vi "PLC.vi"() -> ()   [LabVIEW 2016]
doc: "Sound Analyzer queued state machine"
uses:
  PLC.Data.ctl
  PLC.Data.Status.ctl
  PLC.State.ctl
  PLC.Data.Sets.ctl
  LowLevel/PLC.DataBlock.PCstatus.ctl
  LowLevel/PLC.DataBlock.PCstatus.General.ctl
  LowLevel/PLC.DataBlock.PCstatus.Station.ctl
  LowLevel/PLC.DataBlock.PLCstatus.ctl
  LowLevel/PLC.DataBlock.PLCstatus.General.ctl
  LowLevel/PLC.DataBlock.PLCstatus.Station.ctl
  PLC.Action.ctl
  Tools/CitTemplate/citTemplate.errData.ctl
  Tools/EventLog/EventLog.EventSource.ctl
  PLC.CheckStatusReassembly.ctl
  Database/Database.Global.vi
  PLC.Global.vi
panel:
  out "action":T1=enum."-- PLC --"
  out "error.action":string
  out "error":errorcluster
  out "Data":T2={"Status"={"Idx"=0, "ConnRef"=0, "State"=enum."Off", "LiveBitTimer"=timestamp(0 s since 1904-01-01)}, "Sets"={"Enable"=FALSE, "IP"="", "Rack"=0, "Slot"=10000, "LifeBitTimer_s"=0.0, "DataBlockAddr_PCStatus"=0, "DataBlockAddr_PLCStatus"=1, "DataBlockAddr_PLCNewData"=[], "DataBlockSize_PLCNewData"=[], "DataBlockAddr_PLCChangeOver"=[], "DataBlockSize_PLCChangeOver"=[], "DataBlockAddr_PCChangeOver"=[], "DataBlockAddr_PLCCheckStatus"=[], "DataBlockSize_PLCCheckStatus"=[], "DataBlockAddr_PCCheckStatus"=[]}, "PCstatus"={"General"={"LifeBit"=FALSE, "DbRun"=FALSE}, "Stations"=[]}, "PLCstatus"={"General"={"LifeBit"=FALSE}, "Stations"=[]}}
  out "_loop":i32(ring)=4
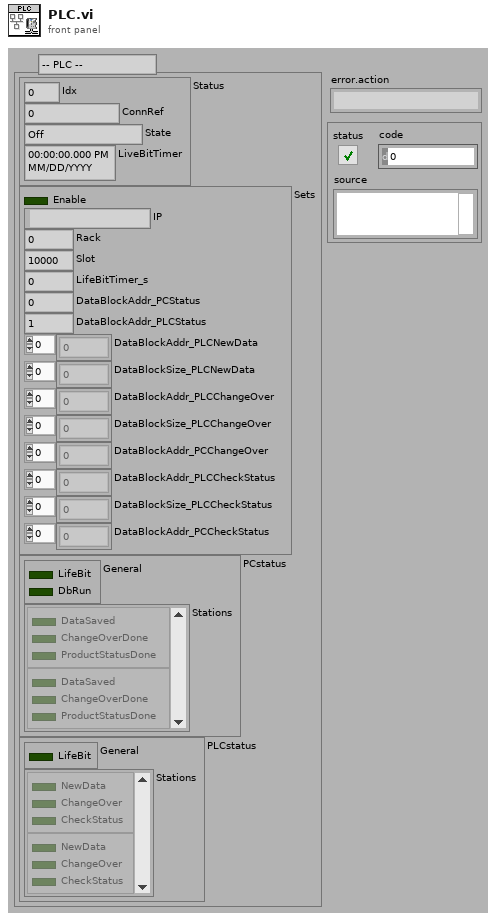
[diagram p1: front panel]
types:
  T1 = typedef "PLC.Action.ctl" = enum32{"idle", "constructor", "destructor", "-- PLC --", "Setup", "NewData", "ChangeOver", "CheckStatus", "Reasembly"}
  T2 = typedef "PLC.Data.ctl" = cluster{"Status":T3, "Sets":T5, "PCstatus":T6, "PLCstatus":T9}
  T3 = typedef "PLC.Data.Status.ctl" = cluster{"Idx":i32, "ConnRef":u64, "State":T4, "LiveBitTimer":timestamp}
  T4 = typedef "PLC.State.ctl" = enum32{"Off", "Error", "Idle", "Run"}
  T5 = typedef "PLC.Data.Sets.ctl" = cluster{"Enable":bool, "IP":string, "Rack":i32, "Slot":i32, "LifeBitTimer_s":dbl, "DataBlockAddr_PCStatus":i32, "DataBlockAddr_PLCStatus":i32, "DataBlockAddr_PLCNewData":i32[], "DataBlockSize_PLCNewData":i32[], "DataBlockAddr_PLCChangeOver":i32[], "DataBlockSize_PLCChangeOver":i32[], "DataBlockAddr_PCChangeOver":i32[], "DataBlockAddr_PLCCheckStatus":i32[], "DataBlockSize_PLCCheckStatus":i32[], "DataBlockAddr_PCCheckStatus":i32[]}
  T6 = typedef "PLC.DataBlock.PCstatus.ctl" = cluster{"General":T7, "Stations":T8[]}
  T7 = typedef "PLC.DataBlock.PCstatus.General.ctl" = cluster{"LifeBit":bool, "DbRun":bool}
  T8 = typedef "PLC.DataBlock.PCstatus.Station.ctl" = cluster{"DataSaved":bool, "ChangeOverDone":bool, "ProductStatusDone":bool}
  T9 = typedef "PLC.DataBlock.PLCstatus.ctl" = cluster{"General":T10, "Stations":T11[]}
  T10 = typedef "PLC.DataBlock.PLCstatus.General.ctl" = cluster{"LifeBit":bool}
  T11 = typedef "PLC.DataBlock.PLCstatus.Station.ctl" = cluster{"NewData":bool, "ChangeOver":bool, "CheckStatus":bool}
  T12 = typedef "EventLog.EventSource.ctl" = enum16{"All", "Gui", "Cache", "PLC1", "PLC2", "PLC3", "DB", "DB01", "DB02", "DB03", "DB04", "DB05", "DB06", "DB07", "DB08", "DB09", "DB10", "DB11", "DB12", "DB13", "DB14", "DB15", "DB16"}
  T13 = typedef "citTemplate.errData.ctl" = cluster{"ts":timestamp, "src":T12, "instance":i32, "action":string, "error":errorcluster, "unconfirmed":bool}
  T14 = typedef "PLC.CheckStatusReassembly.ctl" = cluster{"Ref":string, "Serial":string, "Station":string}
  T15 = typedef "citTemplate.notifierHandle.ctl" = refnum<notifier>
  T16 = typedef "Database.Handler.Data.Status.ctl" = cluster{"Run":bool, "Handle":i32, "ConnTS":timestamp, "DbTime":timestamp, "DbTimeOffset":dbl}
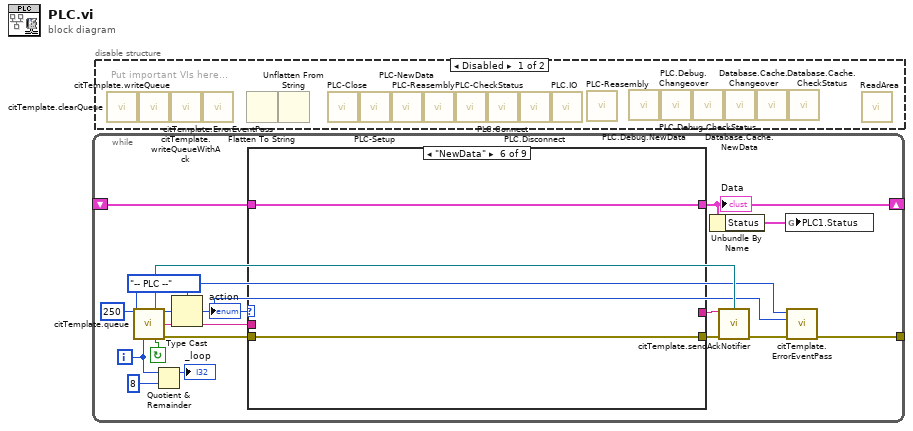
[diagram p0: block diagram]
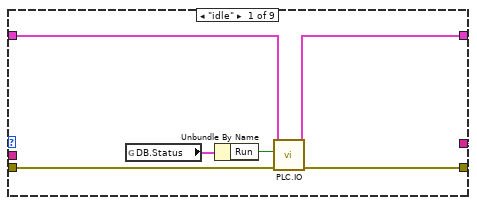
[diagram p2: hidden frame]
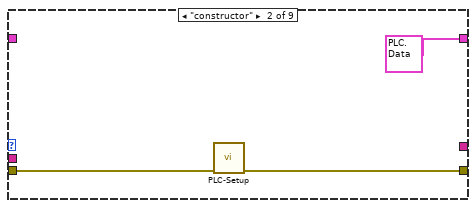
[diagram p3: hidden frame]
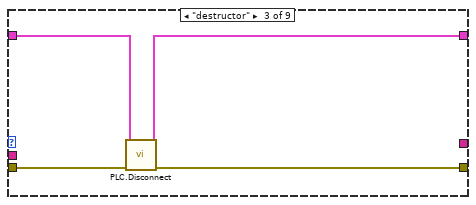
[diagram p4: hidden frame]
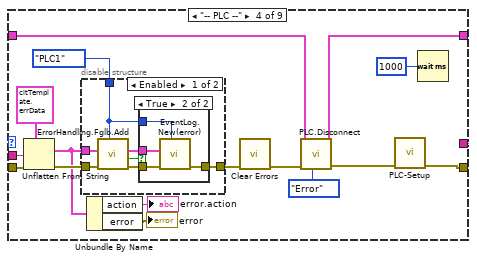
[diagram p5: hidden frame]
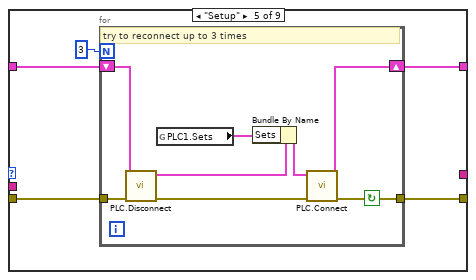
[diagram p8: hidden frame]
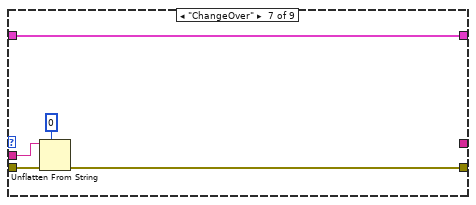
[diagram p9: hidden frame]
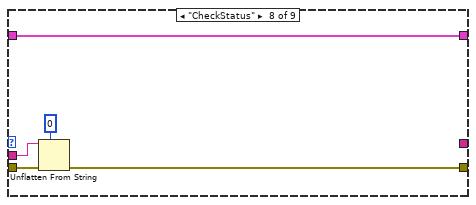
[diagram p10: hidden frame]
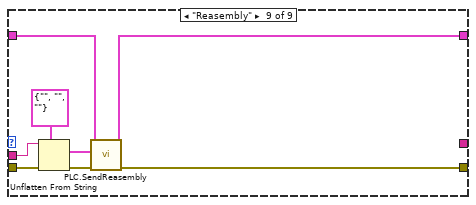
[diagram p11: hidden frame]
diagram:
  n1 = while {
    tunnel: [w7] -> _
    shift-right: [w4] -> _
    shift-left: _ -> [w5]
    i -> [w9]
    stop <- w14 continue-if-true
    w3 = PLC.Action."-- PLC --" ("Action")
    n2 = call "citTemplate.queue.vi"("ms timeout (250 ms)"=250, "event enum"=w3, "iteration (-1)"=w9) -> ("notifierHandle out"=w13:T15, "event out"=w17:u32, "(flatten) data out"=w16:string, "continue"=w14:bool, "error out"=w15:errorcluster)  [unwired: 2 in, 6 out]
    n3 = Quotient & Remainder(x=w9, y=8) -> (x-y*floor(x/y)=→"_loop":i32)  [unwired: 1 out]
    n4 = Type Cast(type=w3, x=w17) -> (*(type *) &x=w8:T1)
    "action" <- w8
    n5 = case shown="\"Reasembly\"" w8 {
      tunnel: w16 -> [_ _ _ w40 _ _ w78 w83 w92]
      tunnel: w15 -> [w22 w27 w31 w41 w65 w74 w79 w84 w93]
      tunnel: ["" _ _ "" _ _ _ _ _] -> w12
      tunnel: [w21 w26 w30 w36 w64 w74 w76 w81 w86] -> w2
      tunnel: [w20 T2 {"Status"={"Idx"=0, "ConnRef"=0, "State"=enum."Off", "LiveBitTimer"=timestamp(0 s since 1904-01-01)}, "Sets"={"Enable"=FALSE, "IP"="", "Rack"=0, "Slot"=10000, "LifeBitTimer_s"=0.0, "DataBlockAddr_PCStatus"=0, "DataBlockAddr_PLCStatus"=0, "DataBlockAddr_PLCNewData"=[], "DataBlockSize_PLCNewData"=[], "DataBlockAddr_PLCChangeOver"=[], "DataBlockSize_PLCChangeOver"=[], "DataBlockAddr_PCChangeOver"=[], "DataBlockAddr_PLCCheckStatus"=[], "DataBlockSize_PLCCheckStatus"=[], "DataBlockAddr_PCCheckStatus"=[]}, "PCstatus"={"General"={"LifeBit"=FALSE, "DbRun"=FALSE}, "Stations"=[]}, "PLCstatus"={"General"={"LifeBit"=FALSE}, "Stations"=[]}} ("Data") w28 w37 w63 w75 w77 w82 w90] -> w4
      tunnel: w5 -> [w23 _ w29 w38 w62 w75 w77 w82 w91]
      frame "idle" {
        n6 = global read "Database.Global.vi" "DB.Status"() -> (w19:T16)
        n7 = Unbundle By Name(w19) -> ("Run"=w18:bool)
        n8 = call "PLC.IO.vi"("error in"=w22, "DbRun"=w18, "Data_in"=w23) -> ("error out"=w21:errorcluster, "Data_out"=w20:T2)  [unwired: 7 in]
      }
      frame "constructor" {
        n9 = call "PLC-Setup.vi"("error in"=w27) -> ("error out"=w26:errorcluster)  [unwired: 10 in]
      }
      frame "destructor" {
        n10 = call "PLC.Disconnect.vi"("error in (no error)"=w31, "Data"=w29) -> ("error out"=w30:errorcluster, "Data out"=w28:T2)  [unwired: 8 in]
      }
      frame "-- PLC --" {
        n11 = Unflatten From String(type=T13 {"ts"=timestamp(0 s since 1904-01-01), "src"=enum."All", "instance"=0, "action"="", "error"={"status"=FALSE, "code"=0, "source"=""}, "unconfirmed"=FALSE} ("ErrData"), binary string=w40, error in (no error)=w41) -> (value=w44:T13, error out=w45:errorcluster)  [unwired: 2 in, 1 out]
        n12 = disable-structure shown="Enabled" {
          disable-tunnel: w45 -> [w54 w60]
          disable-tunnel: w44 -> [w53 _]
          disable-tunnel: [w52 w60] -> w39
          disable-tunnel: EventLog.EventSource."PLC1" ("Event source") -> [w49 _]
          frame Enabled {
            n13 = call "ErrorHandling.Fglb.Add.vi"("Event source"=w49, "error in (no error)"=w54, "Error in"=w53) -> ("error out"=w51:errorcluster, "changed?"=w50:bool)  [unwired: 7 in]
            n14 = case shown="True" w50 {
              tunnel: [w55 w59] -> w52
              tunnel: w53 -> [_ w58]
              tunnel: w51 -> [w55 w57]
              tunnel: w49 -> [_ w56]
              frame False {
              }
              frame True {
                n15 = call "EventLog.New(error).vi"("Source (All)"=w56, "error in"=w57, "ErrData"=w58) -> ("error out"=w59:errorcluster)  [unwired: 8 in]
              }
            }
          }
          frame Disabled {
          }
        }
        n16 = Unbundle By Name(w44) -> ("action"=→"error.action":string, "error"=→"error":errorcluster)
        n17 = call <vilib>:"Clear Errors.vi"("error in (no error)"=w39) -> ("error out"=w33:errorcluster)  [unwired: 5 in, 1 out]
        n18 = call "PLC.Disconnect.vi"("State (Off)"=PLC.State."Error", "error in (no error)"=w33, "Data"=w38) -> ("error out"=w35:errorcluster, "Data out"=w37:T2)  [unwired: 7 in]
        n19 = call "PLC-Setup.vi"("error in"=w35) -> ("error out"=w36:errorcluster)  [unwired: 10 in]
        n20 = Wait (ms)(milliseconds to wait=u32 1000) -> ()  [unwired: 1 out]
      }
      frame "Setup" {
        n21 = for {
          N: 3 -> [_]
          tunnel: w65 -> [w73]
          tunnel: [w66] -> w64
          shift-right: [w71] -> w63
          shift-left: w62 -> [w70]
          stop <- w66 continue-if-true
          # "try to reconnect up to 3 times"
          n22 = call "PLC.Disconnect.vi"("error in (no error)"=w73, "Data"=w70) -> ("error out"=w72:errorcluster, "Data out"=w68:T2)  [unwired: 8 in]
          n23 = global read "PLC.Global.vi" "PLC1.Sets"() -> (w69:T5)
          n24 = Bundle By Name(cluster=w68, "Sets"=w69) -> (w67:T2)
          n25 = call "PLC.Connect.vi"("error in (no error)"=w72, "Data"=w67) -> ("error out"=w66:errorcluster, "Data out"=w71:T2)  [unwired: 8 in]
        }
      }
      frame "NewData" {
      }
      frame "ChangeOver" {
        n26 = Unflatten From String(type=0 ("Slot"), binary string=w78, error in (no error)=w79) -> (error out=w76:errorcluster)  [unwired: 2 in, 2 out]
      }
      frame "CheckStatus" {
        n27 = Unflatten From String(type=0 ("Slot"), binary string=w83, error in (no error)=w84) -> (error out=w81:errorcluster)  [unwired: 2 in, 2 out]
      }
      frame "Reasembly" {
        n28 = Unflatten From String(type=T14 {"Ref"="", "Serial"="", "Station"=""} ("Cluster"), binary string=w92, error in (no error)=w93) -> (value=w88:T14, error out=w87:errorcluster)  [unwired: 2 in, 1 out]
        n29 = call "PLC.SendReasembly.vi"("error in"=w87, "Reasembly data"=w88, "Data_in"=w91) -> ("error out"=w86:errorcluster, "Data out"=w90:T2)  [unwired: 6 in, 1 out]
      }
    }
    "Data" <- w4
    n30 = Unbundle By Name(w4) -> ("Status"=w1:T3)
    n31 = call "citTemplate.sendAckNotifier.vi"("notification data"=w12, "notifierHandle in"=w13, "error in"=w2) -> ()  [unwired: 13 out]
    n32 = global write "PLC.Global.vi" "PLC1.Status"(w1) -> ()
    n33 = call "citTemplate.ErrorEventPass.vi"("error in"=w2, "action of error"=w8, "event in"=w3) -> ("error out"=w7:errorcluster)  [unwired: 2 in, 6 out]
  }
  n34 = disable-structure shown="Disabled" {
    frame Disabled {
      # "Put important VIs here..."
      n35 = call "citTemplate.clearQueue.vi"() -> ()  [unwired: 14 in, 2 out]
      n36 = call "citTemplate.writeQueue.vi"() -> ()  [unwired: 15 in, 1 out]
      n37 = call "citTemplate.writeQueueWithAck.vi"() -> ()  [unwired: 13 in, 3 out]
      n38 = call "citTemplate.ErrorEventPass.vi"() -> ()  [unwired: 11 in, 1 out]
      n39 = Flatten To String() -> ()  [unwired: 4 in, 3 out]
      n40 = Unflatten From String() -> ()  [unwired: 5 in, 3 out]
      n41 = call "PLC-Close.vi"() -> ()  [unwired: 11 in, 1 out]
      n42 = call "PLC-Setup.vi"() -> ()  [unwired: 11 in, 1 out]
      n43 = call "PLC-NewData.vi"() -> ()  [unwired: 11 in, 1 out]
      n44 = call "PLC-Reasembly.vi"() -> ()  [unwired: 11 in, 1 out]
      n45 = call "PLC-CheckStatus.vi"() -> ()  [unwired: 11 in, 1 out]
      n46 = call "PLC.Connect.vi"() -> ()  [unwired: 10 in, 2 out]
      n47 = call "PLC.Disconnect.vi"() -> ()  [unwired: 10 in, 2 out]
      n48 = call "PLC.IO.vi"() -> ()  [unwired: 10 in, 2 out]
      n49 = call "PLC-Reasembly.vi"() -> ()  [unwired: 11 in, 1 out]
      n50 = call "PLC.Debug.NewData.vi"() -> ()  [unwired: 10 in, 2 out]
      n51 = call "PLC.Debug.Changeover.vi"() -> ()  [unwired: 10 in, 2 out]
      n52 = call "PLC.Debug.CheckStatus.vi"() -> ()  [unwired: 10 in, 2 out]
      n53 = call "Database.Cache.NewData.vi"() -> ()  [unwired: 10 in, 2 out]
      n54 = call "Database.Cache.Changeover.vi"() -> ()  [unwired: 10 in, 2 out]
      n55 = call "Database.Cache.CheckStatus.vi"() -> ()  [unwired: 10 in, 2 out]
      n56 = call "ReadArea.vi"() -> ()  [unwired: 12 in]
    }
    frame Enabled {
    }
  }
